vi "Test Create Empty Map.vi"() -> ()   [LabVIEW 2020]
uses:
  3fe8b586-74ca-49a6-9a94-92f4f5315001.vi
  <vilib>/addons/_JKI Toolkits/Caraya/classes/Assert/Assert Equal Value and Type_Variant.vi
  <vilib>/addons/_JKI Toolkits/Caraya/classes/Assert/Assert Not Equal Value_Variant.vi
  <vilib>/addons/_JKI Toolkits/Caraya/classes/Test/Test.lvclass
  <vilib>/addons/_JKI Toolkits/Caraya/classes/Assert/Assert.lvclass
panel:
  out "error out":errorcluster
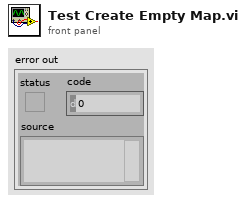
[diagram p1: front panel]
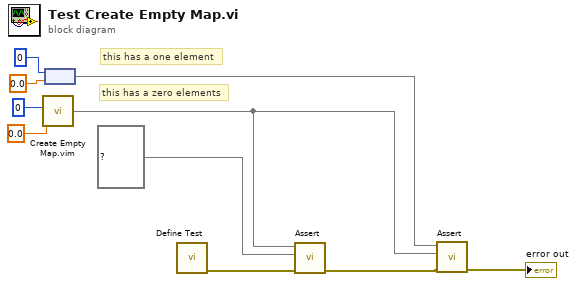
[diagram p0: block diagram]
diagram:
  # "this has a zero elements"
  # "this has a one element"
  n1 = call "Create Empty Map.vim"("value type"=0.0, "key type"=0) -> ("empty map"=w2:map{i32, dbl})  [unwired: 8 in]
  n2 = node ("Build Map")(0, 0.0) -> (w1:map{i32, dbl})
  n3 = call <vilib>:"Define Test.vi"() -> ("error out"=w10:errorcluster)  [unwired: 11 in]
  n4 = call-poly <vilib>:"Assert.vi"("error in (no error)"=w10, "Y"=map{i32, dbl} {} ("empty map"), "X"=w2) -> ("error out"=w4:errorcluster)  [unwired: 8 in]
  n5 = call-poly <vilib>:"Assert.vi"("error in (no error)"=w4, "Y"=w2, "X"=w1) -> ("error out"=→"error out":errorcluster)  [unwired: 8 in]
